vi "kvCanSetStdBusParams.vi"(2 "error in (no error)":errorcluster, 3 "Standard CAN Baud Rate":i32(ring) items=["Classic 1M", "Classic 500K", "Classic 250K", "Classic 125K", "Classic 100K", "Classic 62K", "Classic 50K", "Classic 83K", "FD 500K ", "FD 1M", "FD 2M", "FD 4M", "FD 8M"], 4 "Channel Handle (input only)":i32) -> (0 "error out":errorcluster, 1 "Channel Handle (ouput only)":i32)   [LabVIEW 2022 SP3]
doc: "This function sets the bus timing parameters for the specified CAN controller"
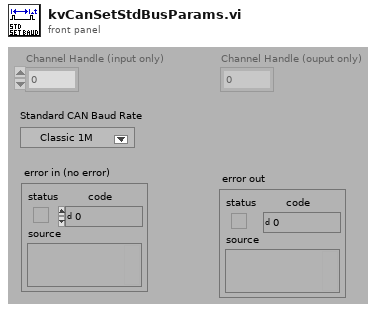
[diagram p1: front panel]
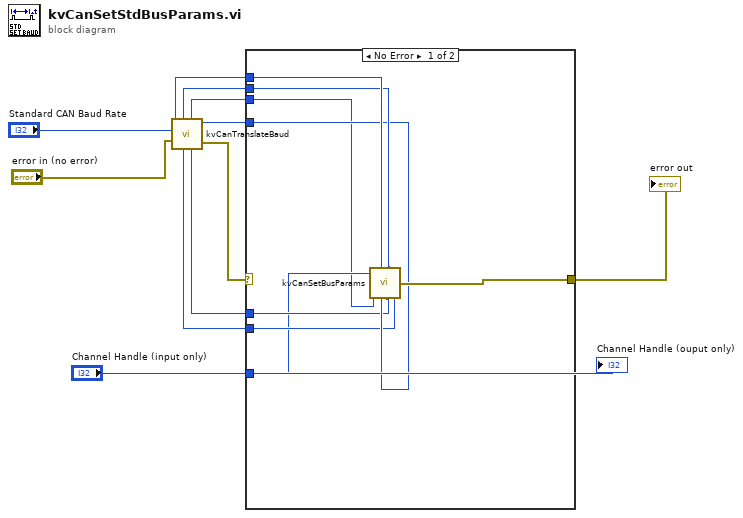
[diagram p0: block diagram]
diagram:
  n1 = call "kvCanTranslateBaud.vi"("error in (no error)"="error in (no error)", "Baud Rate"="Standard CAN Baud Rate") -> ("Sync Mode"=w3:u32, "Number of Sampling Points"=w4:u32, "error out"=w10:errorcluster, "CAN Bus Frequency"=w8:u32, "Time Segment 1"=w7:u32, "Time Segment 2"=w6:u32, "Synchronization Jump Width"=w5:u32)
  n2 = case shown="No Error" w10 {
    selector: w10 -> [_ w20]
    tunnel: [w19 w20] -> w9
    tunnel: w8 -> [w18 _]
    tunnel: w7 -> [w17 _]
    tunnel: w6 -> [w12 _]
    tunnel: w5 -> [w16 _]
    tunnel: w4 -> [w15 _]
    tunnel: w3 -> [w14 _]
    tunnel: "Channel Handle (input only)" -> [w13 _]
    frame No Error {
      n3 = call "kvCanSetBusParams.vi"("Channel Handle (input only)"=w13, "CAN Bus Frequency"=w18, "Time Segment 2"=w12, "Synchronization Jump Width"=w16, "Time Segment 1"=w17, "Number of Sampling Points"=w15, "Sync Mode"=w14) -> ("error out"=w19:errorcluster)  [unwired: 1 in, 1 out]
    }
    frame Error {
    }
  }
  "error out" <- w9
  "Channel Handle (ouput only)" <- "Channel Handle (input only)"
